vi "hmi_initialize.vi"(7 "hmi_references":T1, 8 "error in (no error)":errorcluster) -> (0 "error out":errorcluster)   [LabVIEW 2015, in "lv-build-interface.lvlib"]
uses:
  lv-build-interface.lvlib
  _controls/hmi_references.ctl
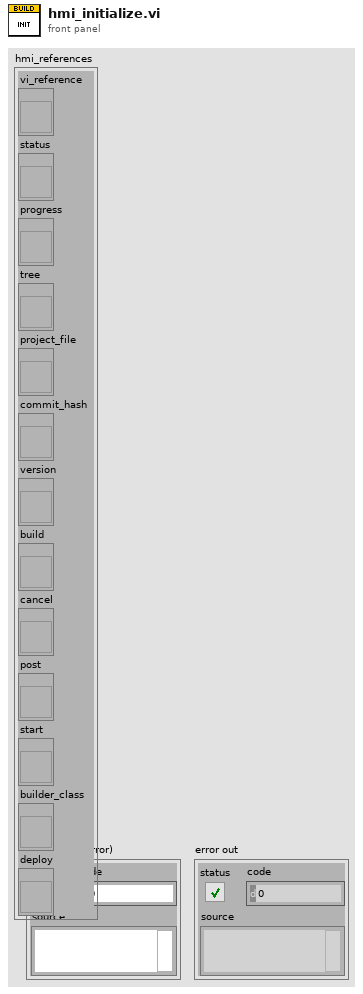
[diagram p1: front panel]
types:
  T1 = typedef "lv-build-interface.lvlib/hmi_references.ctl" = cluster{"vi_reference":refnum<vi>, "status":refnum<vi>, "progress":refnum<vi>, "tree":refnum<vi>, "project_file":refnum<vi>, "commit_hash":refnum<vi>, "version":refnum<vi>, "build":refnum<vi>, "cancel":refnum<vi>, "post":refnum<vi>, "start":refnum<vi>, "builder_class":refnum<vi>, "deploy":refnum<vi>}
  T2 = enum8{"Enabled", "Disabled", "Disabled and Grayed Out"}
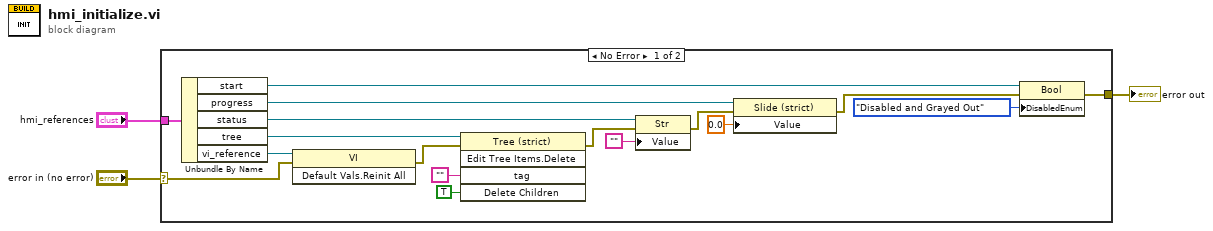
[diagram p0: block diagram]
diagram:
  n1 = case shown="No Error" "error in (no error)" {
    selector: "error in (no error)" -> [w5 w21]
    tunnel: [w4 w21] -> w2
    tunnel: "hmi_references" -> [w20 _]
    frame No Error {
      n2 = Unbundle By Name(w20) -> ("start"=w9:refnum<vi>, "progress"=w15:refnum<vi>, "status"=w16:refnum<vi>, "tree"=w19:refnum<vi>, "vi_reference"=w6:refnum<vi>)
      n3 = invoke class="VI" method="Default Vals.Reinit All"(reference=w6, error in=w5) -> (error out=w10:errorcluster)  [unwired: 1 in, 2 out]
      n4 = invoke class="Tree (strict)" method="Edit Tree Items.Delete"(reference=w19, error in=w10, "tag"="", "Delete Children"=TRUE ("Delete Children?")) -> (error out=w14:errorcluster)  [unwired: 1 in, 4 out]
      n5 = property class="Str"(reference=w16, error in=w14, "Value"="") -> (error out=w13:errorcluster)  [unwired: 1 out]
      n6 = property class="Slide (strict)"(reference=w15, error in=w13, "Value"=0.0) -> (error out=w8:errorcluster)  [unwired: 1 out]
      n7 = property class="Bool"(reference=w9, error in=w8, "DisabledEnum"=T2."Disabled and Grayed Out" ("Disabled")) -> (error out=w4:errorcluster)  [unwired: 1 out]
    }
    frame Error {
    }
  }
  "error out" <- w2
